vi "Connect.vi"(8 "error in":errorcluster, 11 "69X_79X in":refnum<class "69X_79X.lvclass">) -> (0 "error out":errorcluster, 3 "69X_79X out":refnum<class "69X_79X.lvclass">)   [LabVIEW 2019, in "69X_79X.lvlib" / "69X_79X.lvclass"]
uses:
  Library/69X_79X.lvclass
  C:/Users/Public/Documents/Development/builds/Instruments/Instruments.lvlibp/Library/Instruments.lvclass
  Library/69X_79X.lvclass/69X_79X.ctl
  builds/Instruments/Instruments.lvlibp/Accessors/Read Resource.vi
  <instrlib>/Agilent N6900 N7900 Series/Agilent N6900 N7900 Series.lvlib
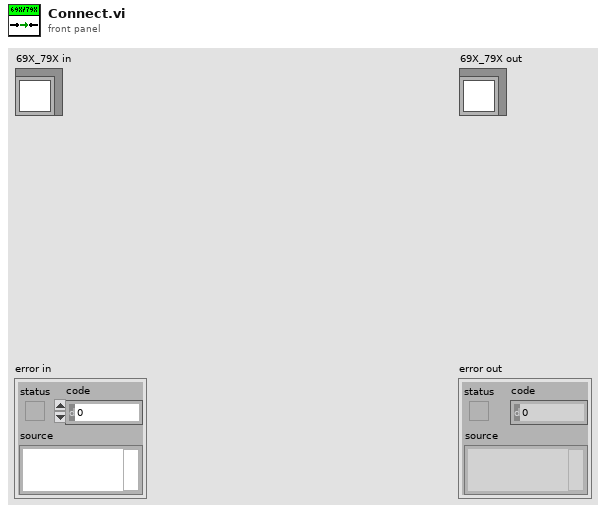
[diagram p1: front panel]
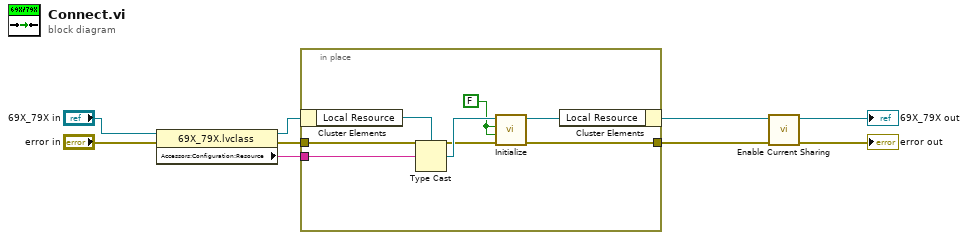
[diagram p0: block diagram]
diagram:
  n1 = property class="69X_79X.lvclass"(reference="69X_79X in", error in="error in") -> (reference out=w4:refnum<class "69X_79X.lvclass">, error out=w3:errorcluster, "Accessors:Configuration:Resource"=w5:string)
  n2 = in-place {
    in-place-border: w5 -> [w15]
    in-place-border: w3 -> [w12]
    in-place-border: [w10] -> w9
    w11 = FALSE ("ID Query (True)")
    n3 = in-place-cluster #1(w4) -> ("Local Resource"=w16:refnum<visa-resource-name>)
    n4 = Type Cast(type=w16, x=w15) -> (*(type *) &x=w14:refnum<visa-resource-name>)
    n5 = call <instrlib>:"Initialize.vi"("error in (no error)"=w12, "Reset (True)"=w11, "ID Query (True)"=w11, "VISA resource name"=w14) -> ("error out"=w10:errorcluster, "VISA resource name out"=w13:refnum<visa-resource-name>)  [unwired: 6 in]
    n6 = in-place-cluster #1("Local Resource"=w13) -> (w8:refnum<class "69X_79X.lvclass">)
  }
  n7 = call "Enable Current Sharing.vi"("error in (no error)"=w9, "69X_79X in"=w8) -> ("error out"=→"error out":errorcluster, "69X_79X out"=→"69X_79X out":refnum<class "69X_79X.lvclass">)  [unwired: 8 in]
